vi "Set Resolution.vi"(0 "video in":refnum<class "MSC Video.lvclass">, 1 "Resolution":T1, 5 "error in (no error)":errorcluster) -> (14 "video out":refnum<class "MSC Video.lvclass">, 15 "Resolution out":T1, 19 "error out":errorcluster)   [LabVIEW 2014, in "MSC Video.lvclass"]
doc: "Sets the camera stream width and height to the selected value.\nIf the value cant be set correctly, it is tried to coerce it to the nearest possible value."
uses:
  MSC Video.lvclass
  MSC Image_class/controls/Size.ctl
  controls/Stream Property.ctl
  MSC Image_class/MSC Image.lvclass
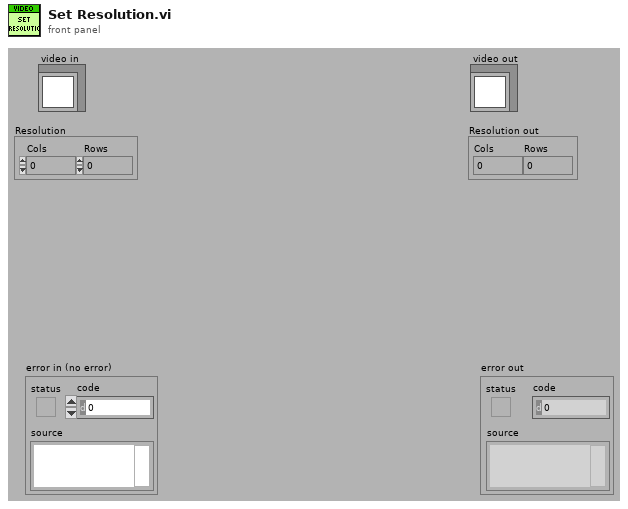
[diagram p1: front panel]
types:
  T1 = typedef "MSC Image.lvclass/Size.ctl" = cluster{"Cols":i32, "Rows":i32}
  T2 = typedef "MSC Video.lvclass/Stream Property.ctl" = u16
  T3 = cluster{"propertyValue":dbl, "propertyValue":dbl}
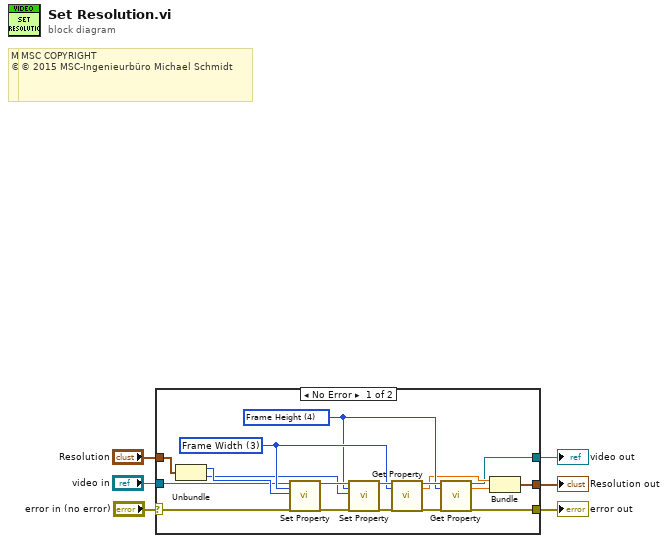
[diagram p0: block diagram]
diagram:
  # "MSC COPYRIGHT\n© 2016 MSC-Ingenieurbüro Michael Schmidt"
  # "MSC COPYRIGHT\n© 2016 MSC-Ingenieurbüro Michael Schmidt"
  # "MSC COPYRIGHT\n© 2015 MSC-Ingenieurbüro Michael Schmidt"
  n1 = case shown="No Error" "error in (no error)" {
    selector: "error in (no error)" -> [w8 w26]
    tunnel: [w7 w26] -> w5
    tunnel: [w9 w25] -> w3
    tunnel: "video in" -> [w10 w25]
    tunnel: "Resolution" -> [w18 _]
    tunnel: [w13 _] -> w1
    frame No Error {
      w16 = T2 4 items=["Position msec", "Position frames", "Position avi ratio", "Frame Width", "Frame Height", "FPS", "Codec", "Frame Count", "Format", "Mode", "Brightness", "Contrast", "Saturation", "Hue", "Gain", "Exposure", "Convert RGB", "White Balance U", "Rectification", "Monochrome", "Sharpness", "Auto Exposure", "Gamma", "Temperature", "Trigger", "Trigger Delay", "White Balance V", "Zoom", "Focus", "Guid", "ISO Speed", "Max DV1394", "Backlight", "Pan", "Tilt", "Rolls", "Iris", "Settings", "Buffersize"] ("Camera Stream Property")
      w17 = T2 3 items=["Position msec", "Position frames", "Position avi ratio", "Frame Width", "Frame Height", "FPS", "Codec", "Frame Count", "Format", "Mode", "Brightness", "Contrast", "Saturation", "Hue", "Gain", "Exposure", "Convert RGB", "White Balance U", "Rectification", "Monochrome", "Sharpness", "Auto Exposure", "Gamma", "Temperature", "Trigger", "Trigger Delay", "White Balance V", "Zoom", "Focus", "Guid", "ISO Speed", "Max DV1394", "Backlight", "Pan", "Tilt", "Rolls", "Iris", "Settings", "Buffersize"] ("Camera Stream Property")
      n2 = Unbundle(w18) -> ("Cols"=w15:i32, "Rows"=w14:i32)
      n3 = call-dynamic "Set Property.vi"("video in"=w10, "Camera Stream Property"=w17, "propertyValue"=w15, "error in (no error)"=w8) -> ("video out"=w20:refnum<class "MSC Video.lvclass">, "error out"=w19:errorcluster)  [unwired: 13 in, 1 out]
      n4 = call-dynamic "Set Property.vi"("video in"=w20, "Camera Stream Property"=w16, "propertyValue"=w14, "error in (no error)"=w19) -> ("video out"=w22:refnum<class "MSC Video.lvclass">, "error out"=w21:errorcluster)  [unwired: 13 in, 1 out]
      n5 = call-dynamic "Get Property.vi"("video in"=w22, "Camera Stream Property"=w17, "error in (no error)"=w21) -> ("video out"=w24:refnum<class "MSC Video.lvclass">, "propertyValue"=w12:dbl, "error out"=w23:errorcluster)  [unwired: 14 in]
      n6 = call-dynamic "Get Property.vi"("video in"=w24, "Camera Stream Property"=w16, "error in (no error)"=w23) -> ("video out"=w9:refnum<class "MSC Video.lvclass">, "propertyValue"=w11:dbl, "error out"=w7:errorcluster)  [unwired: 14 in]
      n7 = Bundle("propertyValue"=w12, "propertyValue"=w11) -> (w13:T3)  [unwired: 1 in]
    }
    frame Error {
    }
  }
  "error out" <- w5
  "video out" <- w3
  "Resolution out" <- w1
